vi "varXNode_Mutate_8_1_0_2.vi"(8 "error in (no error)":errorcluster, 9 "Replies in":string[](array[string]), 10 "Version":T1, 11 "Old State":variant) -> (0 "error out":errorcluster, 1 "Replies out":string[](array[string]), 2 "Version Out":T1, 3 "New State":variant)   [LabVIEW 2017, in "varXNode.xnode"]
uses:
  <vilib>/variable/varXNode.llb/varXNode.xnode
  <vilib>/XNodeSupport/XNodeVersion.ctl
  <vilib>/XNodeSupport/XNodeUShort.ctl
  <vilib>/variable/varXNode.llb/varXNode_old_8_1_0_1.ctl
  <vilib>/variable/Type Descriptor.ctl
  <vilib>/XNodeSupport/NI_XNodeSupport.lvlib
  <vilib>/variable/NI_Variable.lvlib
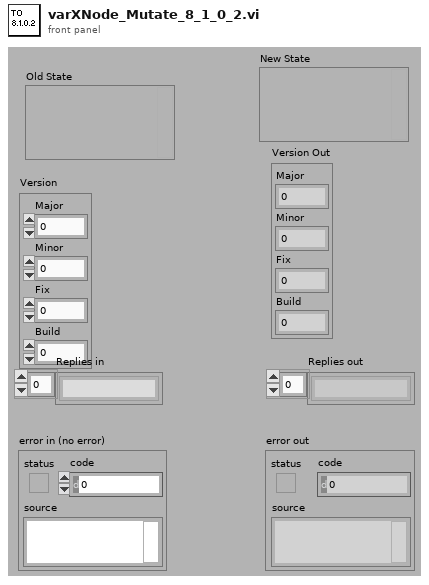
[diagram p1: front panel]
types:
  T1 = typedef "NI_XNodeSupport.lvlib/XNodeVersion.ctl" = cluster{"Major":T2, "Minor":T2, "Fix":T2, "Build":T2}
  T2 = typedef "NI_XNodeSupport.lvlib/XNodeUShort.ctl" = u16
  T3 = typedef "varXNode.xnode/varXNode_old_8_1_0_1.ctl" = cluster{"Write":bool, "ShowTimestamp":bool, "CachedName":string, "CachedTypeDesc":T4, "CachedFeaturePacks":string[], "Custom Rule":string, "ProjectPath":string, "Bad Code":bool, "ContextName":string, "Allow Timestamp":bool, "Generate Code?":bool}
  T4 = typedef "NI_Variable.lvlib/Type Descriptor.ctl" = cluster{"Variant":variant}
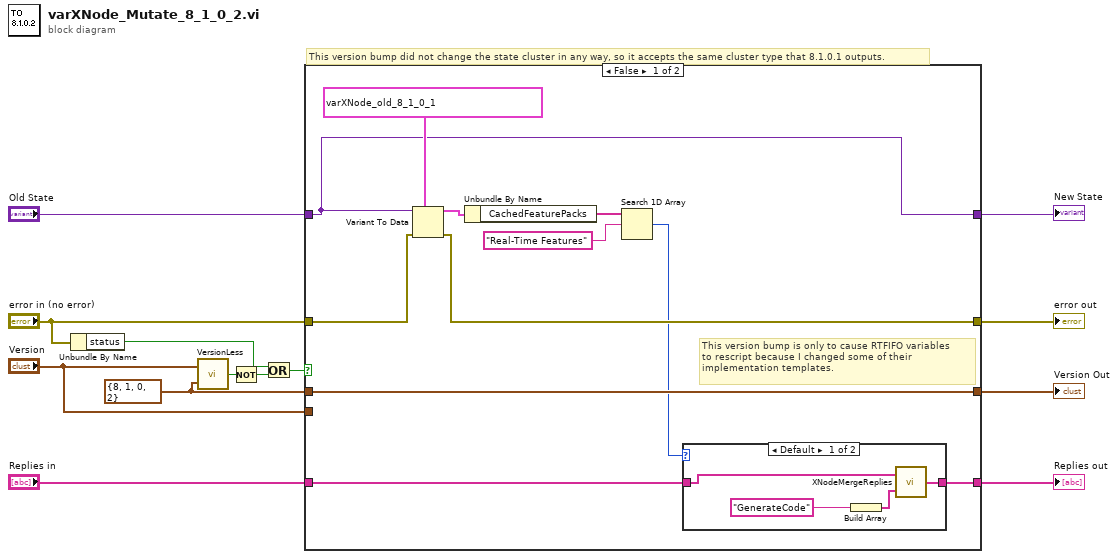
[diagram p0: block diagram]
diagram:
  w12 = T1 {"Major"=8, "Minor"=1, "Fix"=0, "Build"=2} ("y")
  # "This version bump did not change the state cluster in any way, so it accepts the same cluster type that 8.1.0.1 outputs."
  n1 = Unbundle By Name("error in (no error)") -> ("status"=w4:bool)
  n2 = call <vilib>:"VersionLess.vi"("y"=w12, "x"="Version") -> ("x < y?"=w13:bool)
  n3 = Not(x=w13) -> (.not. x?=w3:bool)
  n4 = Or(x=w4, y=w3) -> (x .or. y?=w6:bool)
  n5 = case shown="False" w6 {
    tunnel: w12 -> [w24 _]
    tunnel: [w19 w33] -> w11
    tunnel: "Old State" -> [w19 w33]
    tunnel: [w24 w32] -> w9
    tunnel: "Version" -> [_ w32]
    tunnel: [w22 w31] -> w7
    tunnel: "error in (no error)" -> [w23 w31]
    tunnel: [w14 w30] -> w2
    tunnel: "Replies in" -> [w15 w30]
    frame False {
      # "This version bump is only to cause RTFIFO variables\nto rescript because I changed some of their \nimplementation templates."
      n6 = Variant To Data(error in=w23, type=T3 {"Write"=FALSE, "ShowTimestamp"=FALSE, "CachedName"="", "CachedTypeDesc"={"Variant"=variant}, "CachedFeaturePacks"=[], "Custom Rule"="", "ProjectPath"="", "Bad Code"=FALSE, "ContextName"="", "Allow Timestamp"=FALSE, "Generate Code?"=FALSE} ("State"), Variant=w19) -> (data=w21:T3, error out=w22:errorcluster)
      n7 = Unbundle By Name(w21) -> ("CachedFeaturePacks"=w17:string[])
      n8 = Search 1D Array(1D array=w17, element="Real-Time Features") -> (index of element=w16:i32)  [unwired: 1 in]
      n9 = case shown="Default" w16 {
        tunnel: w15 -> [w28 w29]
        tunnel: [w27 w29] -> w14
        frame Default {
          n10 = Build Array("GenerateCode" ("String")) -> (w26:string[])
          n11 = call <vilib>:"XNodeMergeReplies.vi"("New Replies"=w26, "Old Replies"=w28) -> ("Merged Replies"=w27:string[])
        }
        frame -1 {
        }
      }
    }
    frame True {
      # "Either there was an error in,\nor the version is not less than 8.1.0.2.\nPass input values out."
    }
  }
  "New State" <- w11
  "Version Out" <- w9
  "error out" <- w7
  "Replies out" <- w2
